vi "RS_SMBV100A_NMEA0183_init.vi"(8 "error in":errorcluster) -> (0 "error out":errorcluster, 3 "NMEA0183 Ref":refnum<k7>)   [LabVIEW 2018]
panel:
  out "VI Path":string
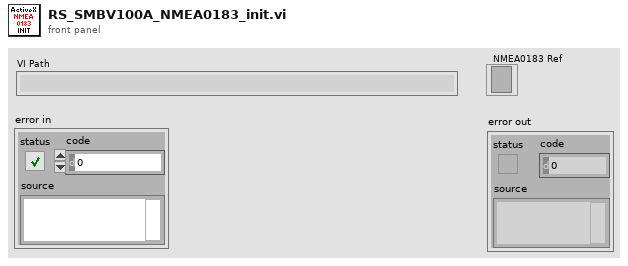
[diagram p1: front panel]
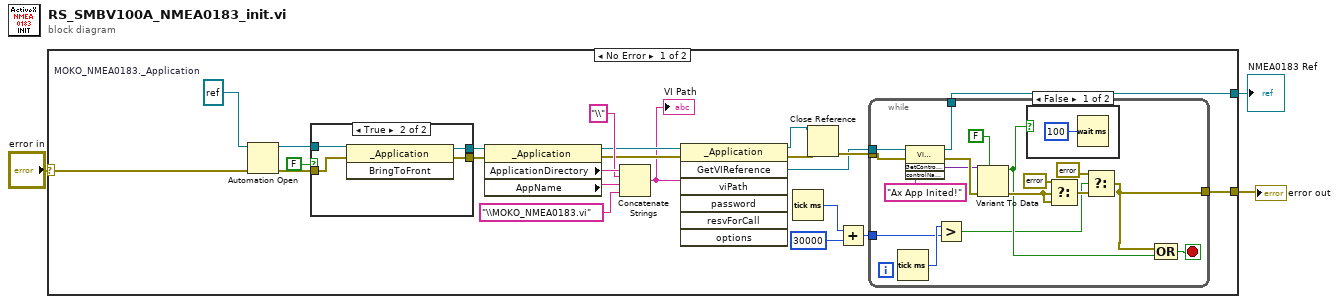
[diagram p0: block diagram]
diagram:
  n1 = case shown="No Error" "error in" {
    selector: "error in" -> [w14 w51]
    tunnel: [w10 w51] -> w3
    tunnel: [w5 _] -> w1
    frame No Error {
      w26 = refnum<k7> refnum  # MOKO_NMEA0183._Application
      n2 = Automation Open(error in (no error)=w14, Automation Refnum=w26) -> (Automation Refnum=w24:refnum<k7>, error out=w25:errorcluster)  [unwired: 2 in]
      n3 = case shown="True" FALSE {
        tunnel: w25 -> [w27 w32]
        tunnel: w24 -> [w28 w31]
        tunnel: [w27 w30] -> w16
        tunnel: [w28 w29] -> w15
        frame False {
        }
        frame True {
          n4 = invoke class="_Application" method="BringToFront"(reference=w31, error in=w32) -> (reference out=w29:refnum<k7>, error out=w30:errorcluster)  [unwired: 1 in, 1 out]
        }
      }
      n5 = property class="_Application"(reference=w15, error in=w16) -> (reference out=w19:refnum<k7>, error out=w18:errorcluster, "ApplicationDirectory"=w23:string, "AppName"=w22:string)
      n6 = Concatenate Strings(w23, "\\" ("string"), w22, "\\MOKO_NMEA0183.vi" ("viPath")) -> (w17:string)
      "VI Path" <- w17
      n7 = invoke class="_Application" method="GetVIReference"(reference=w19, error in=w18, "viPath"=w17) -> (reference out=w11:refnum<k7>, error out=w13:errorcluster, "GetVIReference"=w9:refnum<k7>)  [unwired: 4 in, 4 out]
      n8 = Tick Count (ms)() -> (millisecond timer value=w8:u32)
      n9 = Close Reference(reference=w11, error in (no error)=w13) -> (error out=w12:errorcluster)
      n10 = Add(x=w8, y=u32 30000) -> (x+y=w7:u32)
      n11 = while {
        tunnel: [w46] -> w5
        tunnel: w12 -> [w45]
        tunnel: [w33] -> w10
        tunnel: w9 -> [w43]
        tunnel: w7 -> [w37]
        stop <- w41 stop-if-true
        n12 = Tick Count (ms)() -> (millisecond timer value=w38:u32)
        n13 = invoke class="VirtualInstrument" method="GetControlValue"(reference=w43, error in=w45, "controlName"="Ax App Inited!") -> (reference out=w46:refnum<k7>, error out=w49:errorcluster, "GetControlValue"=w48:variant)  [unwired: 1 in, 1 out]
        n14 = Greater?(x=w38, y=w37) -> (0:w34:bool)
        n15 = Variant To Data(error in=w49, type=FALSE ("status"), Variant=w48) -> (data=w39:bool, error out=w40:errorcluster)
        n16 = case shown="False" w39 {
          frame False {
            n17 = Wait (ms)(milliseconds to wait=u32 100) -> ()  [unwired: 1 out]
          }
          frame True {
          }
        }
        n18 = Select(t=errorcluster {"status"=TRUE, "code"=5005, "source"="Текущий скрипт требует наличия ПО Unitess Vision. Unitess Vision не установлен, либо установлен с ошибками. Переустановите Unitess Vision согласно инструкции по эксплуатации"}, s=w40, f=w40) -> (s? t:f=w36:errorcluster)
        n19 = Select(t=errorcluster {"status"=TRUE, "code"=20486, "source"="Unitess Vision не запускается. Возможно потребуется переустановка ПО согласно инструкции по эксплуатации"} ("error in"), s=w34, f=w36) -> (s? t:f=w33:errorcluster)
        n20 = Compound Arithmetic op=OR(w33, w39) -> (w41:bool)
      }
    }
    frame Error {
    }
  }
  "error out" <- w3
  "NMEA0183 Ref" <- w1
